vi "TestSetProjectConditionalDeactivationValue.vi"(10 "Value":string, 11 "Key":string) -> (0 "Fehler (Ausgang)":errorcluster)   [LabVIEW 2015, in "ConditionalDeactivation.lvlib"]
uses:
  ConditionalDeactivation.lvlib
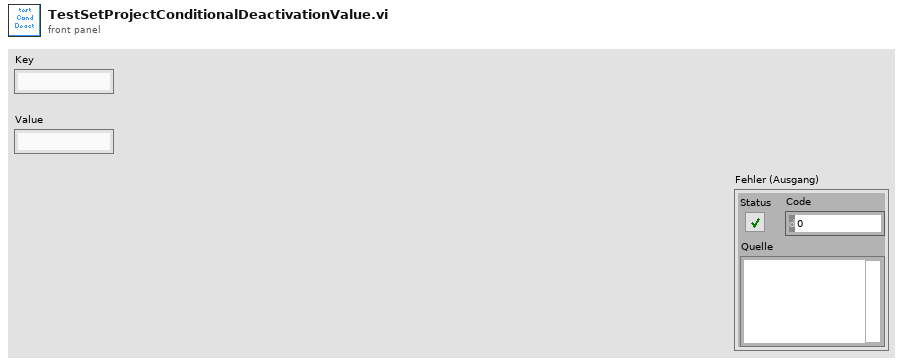
[diagram p1: front panel]
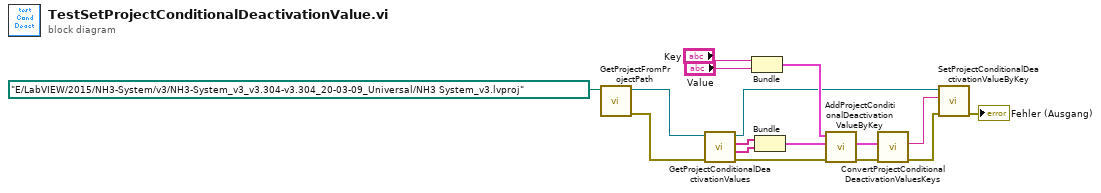
[diagram p0: block diagram]
diagram:
  n1 = call "GetProjectFromProjectPath.vi"("ProjectPfad"=path "E:/LabVIEW/2015/NH3-System/v3/NH3-System_v3_v3.304-v3.304_20-03-09_Universal/NH3 System_v3.lvproj") -> ("Fehler (Ausgang)"=w13:errorcluster, "Projekt Referenz"=w14:refnum<vi>)  [unwired: 9 in]
  n2 = call "GetProjectConditionalDeactivationValues.vi"("Fehler (Eingang, kein Fehler)"=w13, "Projekt Referenz"=w14) -> ("Fehler (Ausgang)"=w12:errorcluster, "Values"=w10:string[], "Keys"=w11:string[], "Projekt Referenz"=w5:refnum<vi>)  [unwired: 5 in, 1 out]
  n3 = Bundle("Key"="Key", "Value"="Value") -> (w6:cluster{"Key":string, "Value":string})  [unwired: 1 in]
  n4 = Bundle("Keys"=w11, "Values"=w10) -> (w9:cluster{"Keys":string[], "Values":string[]})  [unwired: 1 in]
  n5 = call "AddProjectConditionalDeactivationValueByKey.vi"("Fehler (Eingang, kein Fehler)"=w12, "CondDeact"=w9, "Set"=w6) -> ("Fehler (Ausgang)"=w3:errorcluster, "Ausgangs-Cluster"=w4:cluster{string[], string[]})  [unwired: 7 in]
  n6 = call "ConvertProjectConditionalDeactivationValuesKeys.vi"("Fehler (Eingang, kein Fehler)"=w3, "CondDeact"=w4) -> ("Fehler (Ausgang)"=w1:errorcluster, "Tabellen-String"=w2:string)  [unwired: 8 in]
  n7 = call "SetProjectConditionalDeactivationValueByKey.vi"("Fehler (Eingang, kein Fehler)"=w1, "Tabellen-String"=w2, "Projekt Referenz"=w5) -> ("Fehler (Ausgang)"=→"Fehler (Ausgang)":errorcluster)  [unwired: 7 in, 1 out]
